vi "file count function.vi"(8 "error in (no error)":errorcluster, 10 "sub folder name":string, 11 "base path":string) -> (0 "error out":errorcluster, 3 "files found":i32)   [LabVIEW 2015]
panel:
  out "search date":string
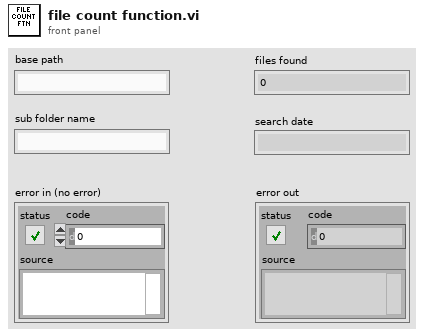
[diagram p1: front panel]
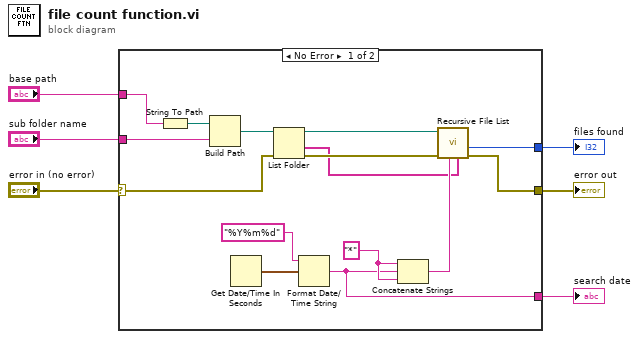
[diagram p0: block diagram]
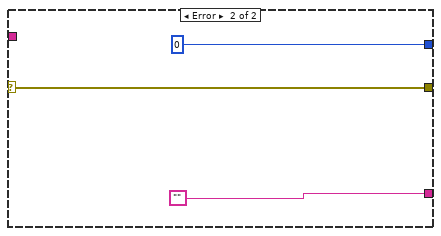
[diagram p2: hidden frame]
diagram:
  n1 = case shown="No Error" "error in (no error)" {
    selector: "error in (no error)" -> [w16 w23]
    tunnel: [w21 0 ("Number of Files")] -> w6
    tunnel: [w11 w23] -> w4
    tunnel: [w12 ""] -> w3
    tunnel: "base path" -> [w9 _]
    tunnel: "sub folder name" -> [w8 _]
    frame No Error {
      w17 = "*" ("string")
      n2 = String To Path(string=w9) -> (path=w10:path)
      n3 = Build Path(base path=w10, name or relative path=w8) -> (appended path=w7:path)
      n4 = Get Date/Time In Seconds() -> (seconds since 1Jan1904=w20:timestamp)
      n5 = List Folder(path=w7, error in=w16) -> (path out=w14:path, folder names=w13:string[], error out=w15:errorcluster)  [unwired: 2 in, 1 out]
      n6 = Format Date/Time String(time format string (%c)="%Y%m%d", seconds (now)=w20) -> (date/time string=w12:string)  [unwired: 1 in]
      n7 = Concatenate Strings(w17, w12, w17) -> (w18:string)
      n8 = call <vilib>:"Recursive File List.vi"("Folders to Exclude"=w13, "pattern"=w18, "error in (no error)"=w15, "Folder Path"=w14) -> ("error out"=w11:errorcluster, "Number of Files"=w21:i32)  [unwired: 3 in, 3 out]
    }
    frame Error {
    }
  }
  "files found" <- w6
  "error out" <- w4
  "search date" <- w3
